vi "Sort 2D Array.vi"(8 "error in (no error)":errorcluster, 9 "Descending (F)":bool, 10 "Priority Columns (0)":i32[](array[numeric])=[0], 11 "Unsorted Array":dbl[][](array[numeric])) -> (0 "error out":errorcluster, 3 "Sorted Array":dbl[][](array[numeric]))   [LabVIEW 2013]
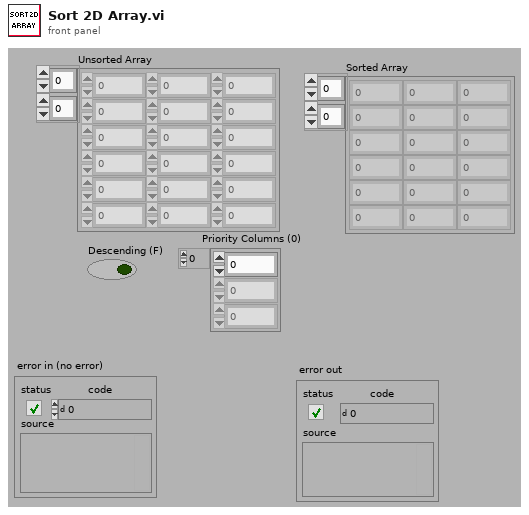
[diagram p1: front panel]
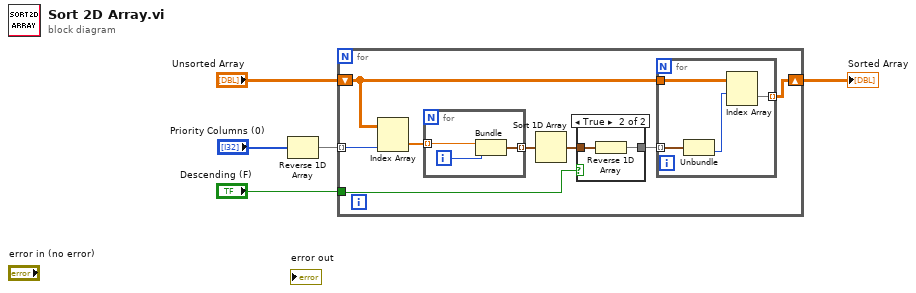
[diagram p0: block diagram]
diagram:
  n1 = Reverse 1D Array(array="Priority Columns (0)") -> (reversed array=w2:i32[])
  n2 = for {
    shift-right: [w7] -> w5
    shift-left: "Unsorted Array" -> [w9]
    tunnel: w2 -> [w6] mode=indexing
    tunnel: "Descending (F)" -> [w8]
    n3 = Index Array(array=w9, index (col)=w6) -> (element=w11:dbl[])  [unwired: 1 in]
    n4 = for {
      tunnel: w11 -> [w21] mode=indexing
      tunnel: [w23] -> w10 mode=indexing
      i -> [w22]
      n5 = Bundle("number: 0 to 1"=w21, w22) -> (w23:cluster{"number: 0 to 1":dbl, i32})  [unwired: 1 out]
    }
    n6 = Sort 1D Array(array=w10) -> (sorted array=w13:cluster{"number: 0 to 1":dbl, i32}[])
    n7 = case shown="True" w8 {
      tunnel: [w14 w15] -> w12
      tunnel: w13 -> [w14 w16]
      frame False {
      }
      frame True {
        n8 = Reverse 1D Array(array=w16) -> (reversed array=w15:cluster{"number: 0 to 1":dbl, i32}[])
      }
    }
    n9 = for {
      tunnel: w12 -> [w20] mode=indexing
      tunnel: w9 -> [w19]
      tunnel: [w17] -> w7 mode=indexing
      n10 = Unbundle(w20) -> (w18:i32)  [unwired: 1 out]
      n11 = Index Array(array=w19, index (row)=w18) -> (element=w17:dbl[])  [unwired: 1 in]
    }
  }
  "Sorted Array" <- w5
